vi "ResetPermission.vi"(8 "error in (no error)":errorcluster, 10 "permission":T1=enum."User", 11 "Person in":refnum<class "Person.lvclass">) -> (0 "error out":errorcluster, 3 "Person out":refnum<class "Person.lvclass">)   [LabVIEW 2014, in "Person.lvclass"]
uses:
  Person.lvclass
  DEF-Permission.ctl
  State_Visitor_class/State_Visitor.lvclass
  State_User_class/State_User.lvclass
  State_Admin_class/State_Admin.lvclass
  Person.lvclass/Person.ctl
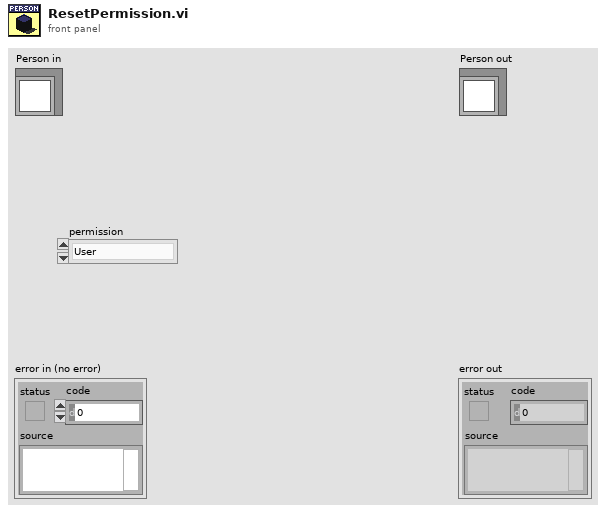
[diagram p1: front panel]
types:
  T1 = typedef "Person.lvclass/DEF-Permission.ctl" = enum16{"Visitor", "User", "Admin"}
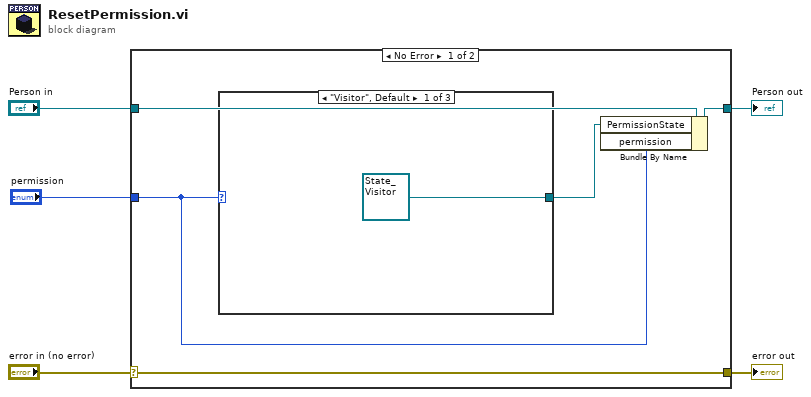
[diagram p0: block diagram]
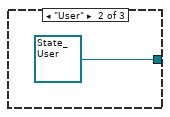
[diagram p2: hidden frame]
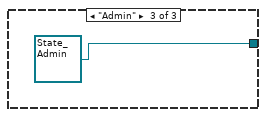
[diagram p3: hidden frame]
diagram:
  n1 = case shown="No Error" "error in (no error)" {
    selector: "error in (no error)" -> [w9 w15]
    tunnel: [w9 w15] -> w4
    tunnel: [w8 w14] -> w2
    tunnel: "Person in" -> [w10 w14]
    tunnel: "permission" -> [w6 _]
    frame No Error {
      n2 = case shown="\"Visitor\", Default" w6 {
        tunnel: [refnum<class "State_Visitor.lvclass"> refnum ("State_Visitor") refnum<class "State_User.lvclass"> refnum ("State_User") refnum<class "State_Admin.lvclass"> refnum ("State_Admin")] -> w7
        frame "Visitor", Default {
        }
        frame "User" {
        }
        frame "Admin" {
        }
      }
      n3 = Bundle By Name(cluster=w10, "PermissionState"=w7, "permission"=w6) -> (w8:refnum<class "Person.lvclass">)
    }
    frame Error {
    }
  }
  "error out" <- w4
  "Person out" <- w2
